vi "Nigel Tamagotchi Full Actor Main.vi"() -> ()   [LabVIEW 2026]
uses:
  1_QMH/Type Defs/Controls Cluster.ctl
  Tamagotchi Full Actor Folder/Tamagotchi Full Actor.lvclass
  C:/Program Files/National Instruments/LabVIEW 2026/vi.lib/ActorFramework/Actor/Actor.lvclass
  Tamagotchi Full Actor Messages/Update Cycles Msg/Update Cycles Msg.lvclass
  C:/Program Files/National Instruments/LabVIEW 2026/vi.lib/ActorFramework/Message/Message.lvclass
  Tamagotchi Full Actor Messages/Update UI Msg/Update UI Msg.lvclass
  <vilib>/ActorFramework/Message Enqueuer/Message Enqueuer.lvclass/Message Enqueuer.ctl
  <vilib>/ActorFramework/Message Enqueuer/Enqueue.vi
  <vilib>/ActorFramework/Stop Msg/Stop Msg.lvclass
  Tamagotchi Full Actor Messages/Feed Msg/Feed Msg.lvclass
  Tamagotchi Full Actor Messages/Clean Msg/Clean Msg.lvclass
  Tamagotchi Full Actor Messages/Sleep Msg/Sleep Msg.lvclass
  Tamagotchi Full Actor Messages/Spaghetti Msg/Spaghetti Msg.lvclass
  Tamagotchi Full Actor Messages/Broken Arrow Msg/Broken Arrow Msg.lvclass
  Tamagotchi Full Actor Messages/Fixed Bug Msg/Fixed Bug Msg.lvclass
  Tamagotchi Full Actor Messages/Launch Hardware Interface Msg/Launch Hardware Interface Msg.lvclass
  <vilib>/ActorFramework/Message Priority Queue/Priority Enqueue.vi
  <vilib>/ActorFramework/Actor/Actor.lvclass
  <vilib>/ActorFramework/Actor Framework.lvlib
panel:
  in  "Launch Hardware Interface":bool
  in  "Stop":bool
  out "Age (cycles)":u32
  out "Mood":string
  out "Cleanliness":i16(slide)=100 scale=0.0..100.0
  out "Energy":i16(slide)=100 scale=0.0..100.0
  out "Hunger":i16(slide) scale=0.0..100.0
  in  "Fixed Bug Button":bool
  in  "Broken Arrow Button":bool
  in  "Spagetti Button":bool
  in  "Sleep Button":bool
  in  "Clean Button":bool
  in  "Feed Button":bool
  out "Pict Ring":u16(ring)
  # "Nigel-gotchi (Full Actor)"
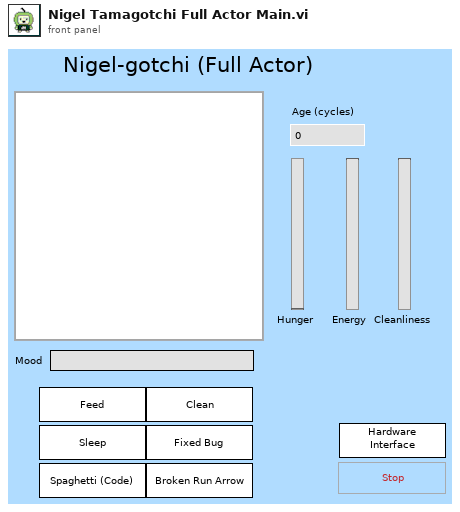
[diagram p1: front panel]
types:
  T1 = typedef "Controls Cluster.ctl" = cluster{"Pict Ring":refnum<vi>, "Mood":refnum<vi>, "Cleanliness":refnum<vi>, "Hunger":refnum<vi>, "Energy":refnum<vi>, "Age (cycles)":refnum<vi>}
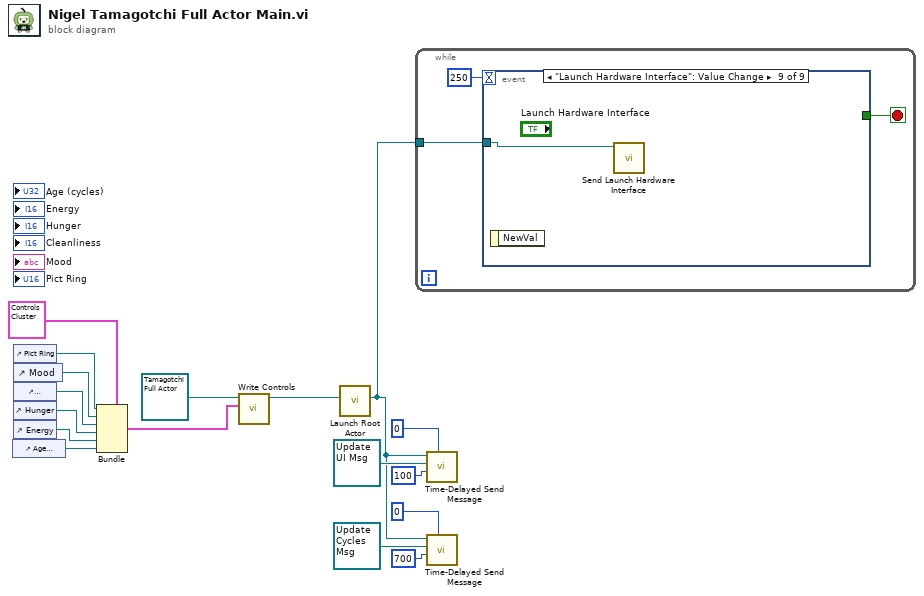
[diagram p0: block diagram]
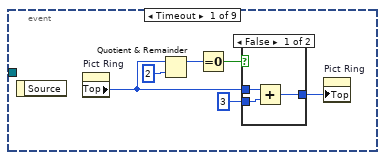
[diagram p2: hidden frame]
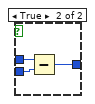
[diagram p3: hidden frame]
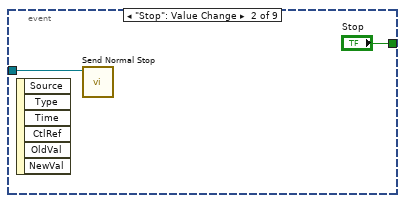
[diagram p4: hidden frame]
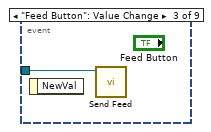
[diagram p5: hidden frame]
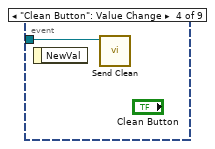
[diagram p6: hidden frame]
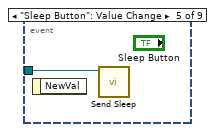
[diagram p7: hidden frame]
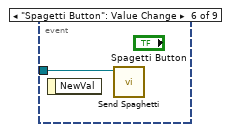
[diagram p8: hidden frame]
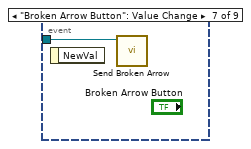
[diagram p9: hidden frame]
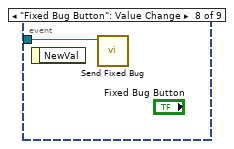
[diagram p10: hidden frame]
diagram:
  n1 = control-ref of="Age (cycles)"() -> (w12:refnum<vi>)
  n2 = control-ref of="Pict Ring"() -> (w17:refnum<vi>)
  n3 = control-ref of="Mood"() -> (w16:refnum<vi>)
  n4 = control-ref of="Cleanliness"() -> (w15:refnum<vi>)
  n5 = control-ref of="Hunger"() -> (w14:refnum<vi>)
  n6 = control-ref of="Energy"() -> (w13:refnum<vi>)
  n7 = Bundle(cluster=T1 {"Pict Ring"=refnum, "Mood"=refnum, "Cleanliness"=refnum, "Hunger"=refnum, "Energy"=refnum, "Age (cycles)"=refnum} ("Controls"), "Pict Ring"=w17, "Mood"=w16, "Cleanliness"=w15, "Hunger"=w14, "Energy"=w13, "Age (cycles)"=w12) -> (w9:T1)
  n8 = call-dynamic "Write Controls.vi"("Controls"=w9, "Nigel Tamagotchi in"=refnum<class "Tamagotchi Full Actor.lvclass"> refnum ("Tamagotchi Full Actor.lvclass")) -> ("Nigel Tamagotchi out"=w1:refnum<class "Tamagotchi Full Actor.lvclass">)  [unwired: 8 in, 1 out]
  n9 = call <vilib>:"Launch Root Actor.vi"("Actor"=w1) -> ("Actor's Enqueuer"=w2:refnum<class "Message Enqueuer.lvclass">)  [unwired: 9 in, 1 out]
  n10 = while {
    tunnel: w2 -> [w18]
    stop <- w20 stop-if-true
    n11 = event shown="[8] \"Launch Hardware Interface\": Value Change" {
      selector: _ -> [_ _ _ _ _ _ _ _ _]
      dyn-events: _ -> [_ _ _ _ _ _ _ _ _]
      timeout: 250 -> [_ _ _ _ _ _ _ _ _]
      tunnel: [_ "Stop" _ _ _ _ _ _ _] -> w20
      tunnel: w18 -> [_ w33 w35 w36 w37 w38 w39 w40 w41]
      event Timeout {
        n12 = event-data() -> ()  [unwired: 1 in, 1 out]
        n13 = property on="Pict Ring" class="Ring (strict)"() -> ("Top"=w25:i32)  [unwired: 2 in, 2 out]
        n14 = Quotient & Remainder(x=w25, y=2) -> (x-y*floor(x/y)=w23:i32)  [unwired: 1 out]
        n15 = Equal To 0?(x=w23) -> (x = 0?=w24:bool)
        n16 = case shown="False" w24 {
          tunnel: w25 -> [w29 w32]
          tunnel: 3 ("y") -> [w28 w31]
          tunnel: [w27 w30] -> w26
          frame False {
            n17 = Add(x=w29, y=w28) -> (x+y=w27:i32)
          }
          frame True {
            n18 = Subtract(x=w32, y=w31) -> (x-y=w30:i32)
          }
        }
        n19 = property on="Pict Ring" class="Ring (strict)"("Top"=w26) -> ()  [unwired: 2 in, 2 out]
      }
      event "Stop": Value Change {
        n20 = event-data() -> ()  [unwired: 1 in, 6 out]
        n21 = call <vilib>:"Send Normal Stop.vi"("Message Enqueuer"=w33) -> ()  [unwired: 10 in, 1 out]
      }
      event "Feed Button": Value Change {
        n22 = event-data() -> ()  [unwired: 1 in, 1 out]
        n23 = call "Send Feed.vi"("Message Enqueuer"=w35) -> ()  [unwired: 9 in, 2 out]
      }
      event "Clean Button": Value Change {
        n24 = event-data() -> ()  [unwired: 1 in, 1 out]
        n25 = call "Send Clean.vi"("Message Enqueuer"=w36) -> ()  [unwired: 9 in, 2 out]
      }
      event "Sleep Button": Value Change {
        n26 = event-data() -> ()  [unwired: 1 in, 1 out]
        n27 = call "Send Sleep.vi"("Message Enqueuer"=w37) -> ()  [unwired: 9 in, 2 out]
      }
      event "Spagetti Button": Value Change {
        n28 = event-data() -> ()  [unwired: 1 in, 1 out]
        n29 = call "Send Spaghetti.vi"("Message Enqueuer"=w38) -> ()  [unwired: 9 in, 2 out]
      }
      event "Broken Arrow Button": Value Change {
        n30 = event-data() -> ()  [unwired: 1 in, 1 out]
        n31 = call "Send Broken Arrow.vi"("Message Enqueuer"=w39) -> ()  [unwired: 9 in, 2 out]
      }
      event "Fixed Bug Button": Value Change {
        n32 = event-data() -> ()  [unwired: 1 in, 1 out]
        n33 = call "Send Fixed Bug.vi"("Message Enqueuer"=w40) -> ()  [unwired: 9 in, 2 out]
      }
      event "Launch Hardware Interface": Value Change {
        n34 = event-data() -> ()  [unwired: 1 in, 1 out]
        n35 = call "Send Launch Hardware Interface.vi"("Message Enqueuer"=w41) -> ()  [unwired: 9 in, 2 out]
      }
    }
  }
  n36 = call <vilib>:"Time-Delayed Send Message.vi"("# Copies (0 = infinite repeat)"=u32 0, "Milliseconds To Wait"=100 ("milliseconds to wait"), "Message"=refnum<class "Update UI Msg.lvclass"> refnum ("Update UI Msg.lvclass"), "Message Enqueuer"=w2) -> ()  [unwired: 6 in, 2 out]
  n37 = call <vilib>:"Time-Delayed Send Message.vi"("# Copies (0 = infinite repeat)"=u32 0, "Milliseconds To Wait"=700 ("milliseconds to wait"), "Message"=refnum<class "Update Cycles Msg.lvclass"> refnum ("Update Cycles Msg.lvclass"), "Message Enqueuer"=w2) -> ()  [unwired: 6 in, 2 out]
